vi "CMI ADS127L21 - Config Sampling Rate.vi"(8 "error in (no error)":errorcluster, 10 "Sampling rate [Hz]":dbl, 11 "session in":T1 {"channels"."Channel" min=1 max=8 step=1; "channels"."Range [Vpk]" items=["±1.65V", "±2V"]}) -> (0 "error out":errorcluster, 3 "session out":T1 {"channels"."Channel" min=1 max=8 step=1; "channels"."Range [Vpk]" items=["±1.65V", "±2V"]})   [LabVIEW 2020]
doc: "Set desired sampling rate."
uses:
  CMI ADS127L21 - Session.ctl
  CMI ADS127L21 - Record Channel.ctl
  CMI ADS127L21 - Input Range.ctl
  CMI ADS127L21 - Input Mode.ctl
  CMI ADS127L21 - Input Impedance.ctl
  CMI ADS127L21 - EXTOUT Mode.ctl
  CMI ADS127L21 - EXTOUT Polarity.ctl
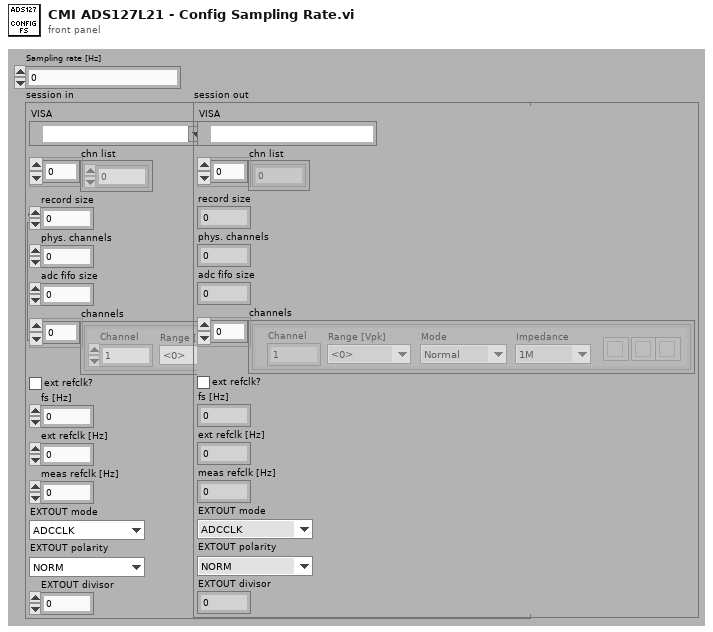
[diagram p1: front panel]
types:
  T1 = typedef "CMI ADS127L21 - Session.ctl" = cluster{"VISA":refnum<visa-resource-name>, "chn list":i32[], "record size":i32, "phys. channels":i32, "adc fifo size":i32, "channels":T2[], "ext refclk?":bool, "fs [Hz]":dbl, "ext refclk [Hz]":dbl, "meas refclk [Hz]":dbl, "EXTOUT mode":T6, "EXTOUT polarity":T7, "EXTOUT divisor":i32}
  T2 = typedef "CMI ADS127L21 - Record Channel.ctl" = cluster{"Range [Vpk]":T3, "Channel":i32, "Mode":T4, "Impedance":T5, "btn clr":bool, "btn up":bool, "btn down":bool}
  T3 = typedef "CMI ADS127L21 - Input Range.ctl" = dbl
  T4 = typedef "CMI ADS127L21 - Input Mode.ctl" = enum16{"Normal", "Inverted", "GND"}
  T5 = typedef "CMI ADS127L21 - Input Impedance.ctl" = enum16{"1M", "1k5"}
  T6 = typedef "CMI ADS127L21 - EXTOUT Mode.ctl" = enum16{"ADCCLK", "REFCLK", "SMPLCLK", "FIRST"}
  T7 = typedef "CMI ADS127L21 - EXTOUT Polarity.ctl" = enum16{"NORM", "INV"}
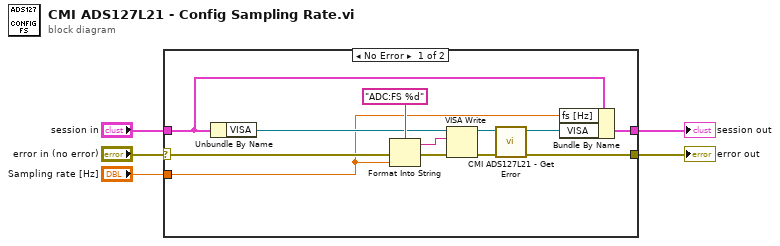
[diagram p0: block diagram]
diagram:
  n1 = case shown="No Error" "error in (no error)" {
    selector: "error in (no error)" -> [w10 w19]
    tunnel: "Sampling rate [Hz]" -> [w6 _]
    tunnel: "session in" -> [w7 w18]
    tunnel: [w8 w18] -> w4
    tunnel: [w11 w19] -> w3
    frame No Error {
      n2 = Unbundle By Name(w7) -> ("VISA"=w9:refnum<visa-resource-name>)
      n3 = Format Into String(format string="ADC:FS %d", error in=w10, w6) -> (resulting string=w13:string, error out=w16:errorcluster)  [unwired: 1 in]
      n4 = VISA Write(VISA resource name=w9, write buffer=w13, error in (no error)=w16) -> (VISA resource name out=w14:refnum<visa-resource-name>, error out=w15:errorcluster)  [unwired: 1 out]
      n5 = call "CMI ADS127L21 - Get Error.vi"("error in (no error)"=w15, "VISA in"=w14) -> ("error out"=w11:errorcluster, "VISA out"=w12:refnum<visa-resource-name>)  [unwired: 8 in]
      n6 = Bundle By Name(cluster=w7, "fs [Hz]"=w6, "VISA"=w12) -> (w8:T1)
    }
    frame Error {
    }
  }
  "error out" <- w3
  "session out" <- w4
